vi "Login.vi"(8 "error in (no error)":errorcluster, 11 "connection reference":T1) -> (0 "error out":errorcluster, 1 "valid?":bool, 2 "userInfo":T2, 3 "connection reference out":T1)   [LabVIEW 2015]
uses:
  <vilib>/addons/database/Connection.llb/Conn ObjectReference.ctl
  <vilib>/Utility/miscctls.llb/LVPointTypeDef.ctl
  <vilib>/addons/database/_DB Variant To Data/Database Variant To Data.xnode
  <vilib>/addons/database/NI_Database_API.lvlib
panel:
  in  "cancelBT":bool
  in  "loginBT":bool
  in  "PASSWORD":string
  in  "USER NAME":string
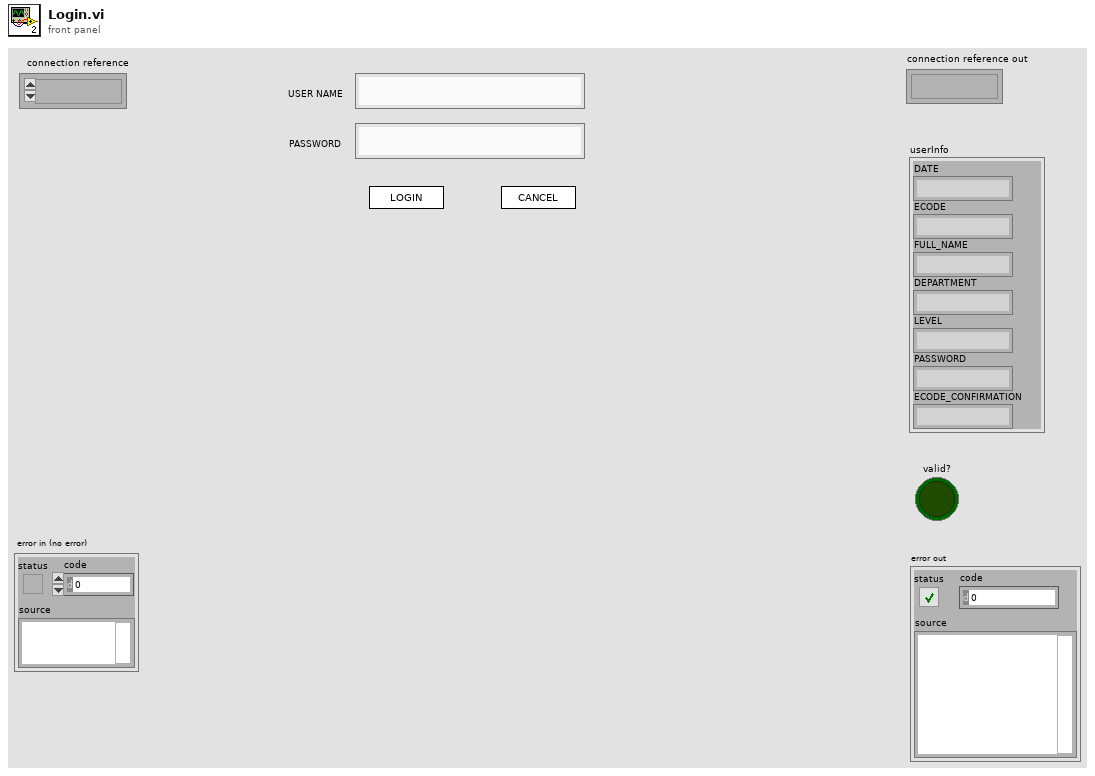
[diagram p1: front panel]
types:
  T1 = typedef "NI_Database_API.lvlib/Conn ObjectReference.ctl" = refnum<k1>
  T2 = cluster{"DATE":string, "ECODE":string, "FULL_NAME":string, "DEPARTMENT":string, "LEVEL":string, "PASSWORD":string, "ECODE_CONFIRMATION":string}
  T3 = typedef "LVPointTypeDef.ctl" = cluster{"Horizontal":i16, "Vertical":i16}
  T4 = cluster{"DATE":string, "ECODE":string, "FULL_NAME":string, "DEPARTMENT":string, "LEVEL":string, "PASSWORD":string, "ECODE_CONFIRMATION":string}[]
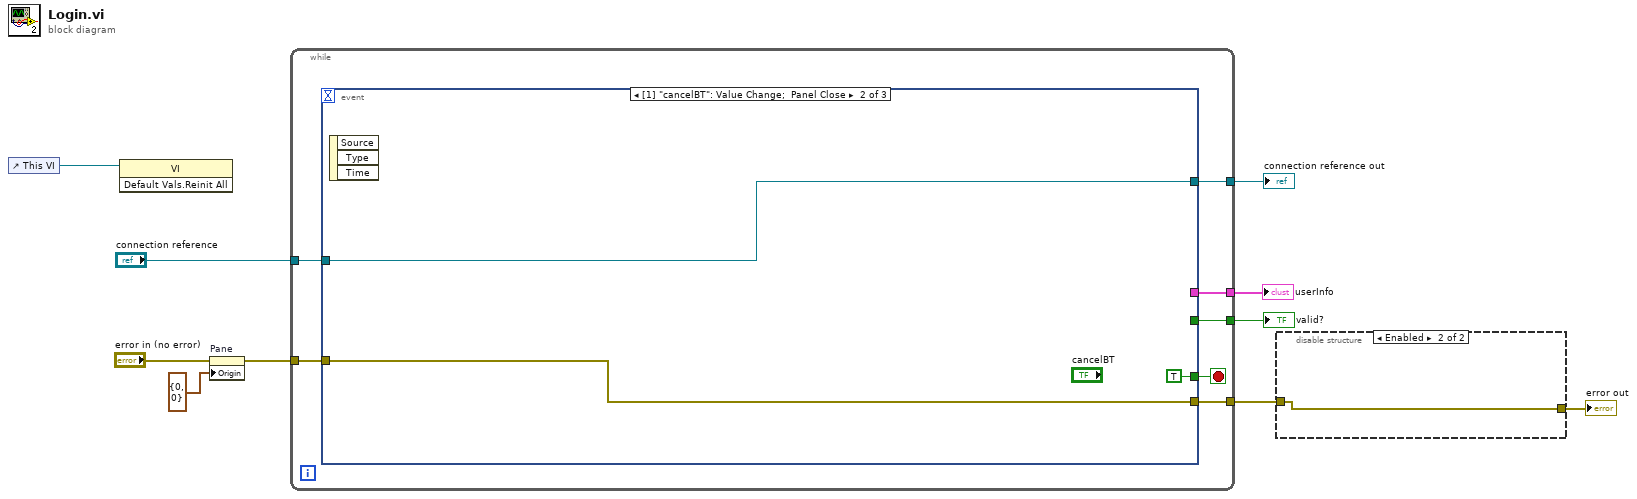
[diagram p0: block diagram]
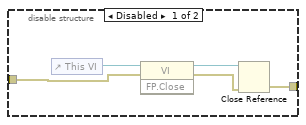
[diagram p2: hidden frame]
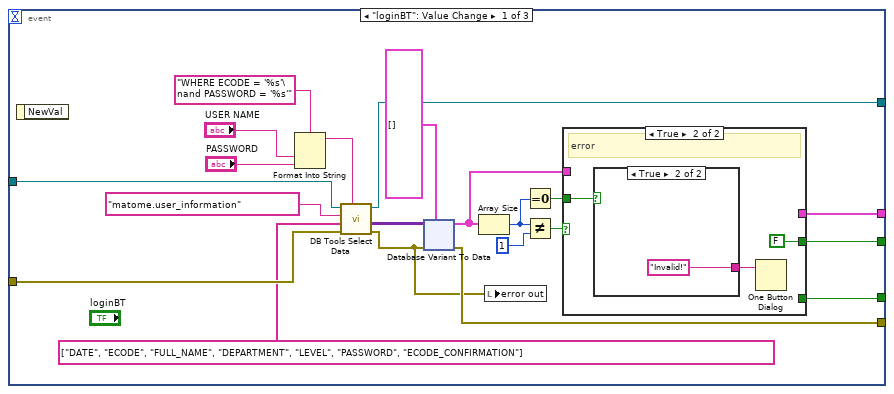
[diagram p3: hidden frame]
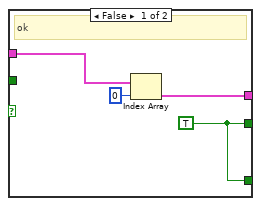
[diagram p4: hidden frame]
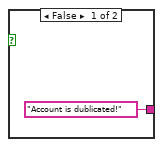
[diagram p5: hidden frame]
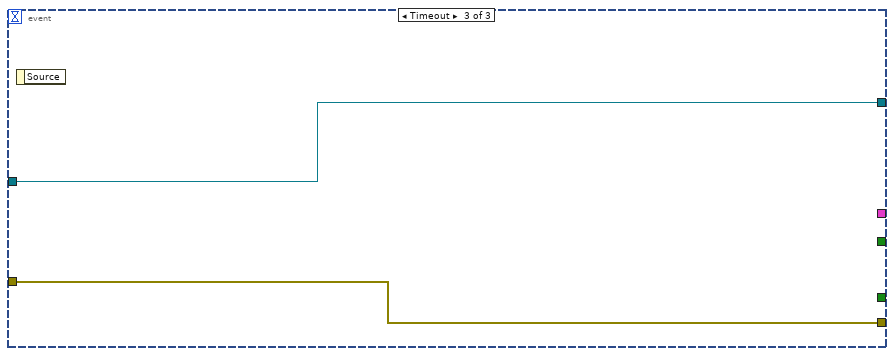
[diagram p6: hidden frame]
diagram:
  n1 = control-ref of="This VI"() -> (w1:refnum<vi>)
  n2 = invoke class="VI" method="Default Vals.Reinit All"(reference=w1) -> ()  [unwired: 2 in, 3 out]
  n3 = property on="Pane" class="Pane"(error in="error in (no error)", "Origin"=T3 {"Horizontal"=0, "Vertical"=0}) -> (error out=w5:errorcluster)  [unwired: 1 in, 1 out]
  n4 = while {
    tunnel: "connection reference" -> [w17]
    tunnel: w5 -> [w16]
    tunnel: [w15] -> w10
    tunnel: [w14] -> w9
    tunnel: [w12] -> w2
    tunnel: [w11] -> w8
    stop <- w13 stop-if-true
    n5 = event shown="[1] \"cancelBT\": Value Change;  Panel Close" {
      selector: _ -> [_ _ _]
      dyn-events: _ -> [_ _ _]
      timeout: _ -> [_ _ _]
      tunnel: w17 -> [w38 w277 w278]
      tunnel: w16 -> [w37 w276 w279]
      tunnel: [w36 _ _] -> w15
      tunnel: [w35 _ _] -> w14
      tunnel: [w32 TRUE _] -> w13
      tunnel: [w34 w276 w279] -> w12
      tunnel: [w33 w277 w278] -> w11
      event "loginBT": Value Change {
        n6 = event-data() -> ()  [unwired: 1 in, 1 out]
        n7 = Format Into String(format string="WHERE ECODE = '%s'\nand PASSWORD = '%s'" ("condition"), "USER NAME", "PASSWORD") -> (resulting string=w26:string)  [unwired: 2 in, 1 out]
        n8 = call <vilib>:"DB Tools Select Data.vi"("condition"=w26, "error in (no error)"=w37, "columns"=string[] ["DATE", "ECODE", "FULL_NAME", "DEPARTMENT", "LEVEL", "PASSWORD", "ECODE_CONFIRMATION"] ("Array"), "table"="matome.user_information", "connection reference"=w38) -> ("error out"=w18:errorcluster, "data"=w28:variant[][], "connection reference out"=w33:T1)  [unwired: 1 in]
        n9 = xnode "Database Variant To Data"("database variant"=w28, "error in (no error)"=w18, "type"=T4 []) -> ("data"=w21:T4, "error out"=w34:errorcluster)
        n10 = Array Size(array=w21) -> (size(s)=w20:i32)
        n11 = local write "error out"(w18) -> ()
        n12 = Equal To 0?(x=w20) -> (x = 0?=w19:bool)
        n13 = Not Equal?(x=w20, y=1) -> (x != y?=w22:bool)
        n14 = case shown="True" w22 {
          tunnel: [w39 FALSE] -> w35
          tunnel: w21 -> [w42 _]
          tunnel: [w40 _] -> w36
          tunnel: w19 -> [_ w44]
          tunnel: [w39 _] -> w32
          frame False {
            w39 = TRUE
            # "ok"
            n15 = Index Array(array=w42, index=0) -> (element=w40:T2)
          }
          frame True {
            # "error"
            n16 = case shown="True" w44 {
              tunnel: ["Account is dublicated!" ("message") "Invalid!" ("message")] -> w43
              frame False {
              }
              frame True {
              }
            }
            n17 = One Button Dialog(message=w43) -> ()  [unwired: 1 in, 1 out]
          }
        }
      }
      event "cancelBT": Value Change; Panel Close {
        n18 = event-data() -> ()  [unwired: 1 in, 3 out]
      }
      event Timeout {
        n19 = event-data() -> ()  [unwired: 1 in, 1 out]
      }
    }
  }
  "userInfo" <- w10
  "valid?" <- w9
  "connection reference out" <- w8
  n20 = disable-structure shown="Enabled" {
    disable-tunnel: [w281 w285] -> w3
    disable-tunnel: w2 -> [w280 w285]
    frame Disabled {
      n21 = control-ref of="This VI"() -> (w284:refnum<vi>)
      n22 = invoke class="VI" method="FP.Close"(reference=w284, error in=w280) -> (reference out=w283:refnum<vi>, error out=w282:errorcluster)  [unwired: 1 in, 1 out]
      n23 = Close Reference(reference=w283, error in (no error)=w282) -> (error out=w281:errorcluster)
    }
    frame Enabled {
    }
  }
  "error out" <- w3
